vi "Error.Case Redirect on Error.vi"(7 "Error Case":string="Done", 10 "error in":errorcluster, 11 "Next Case":string) -> (3 "Next Case Out":string)   [LabVIEW 2018]
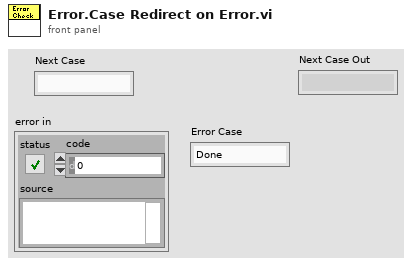
[diagram p1: front panel]
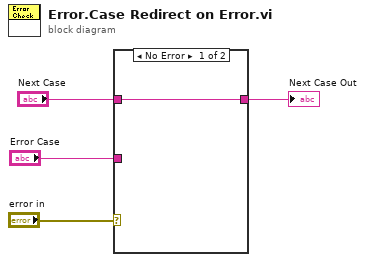
[diagram p0: block diagram]
diagram:
  n1 = case shown="No Error" "error in" {
    tunnel: "Next Case" -> [w5 _]
    tunnel: [w5 w6] -> w2
    tunnel: "Error Case" -> [_ w6]
    frame No Error {
    }
    frame Error {
    }
  }
  "Next Case Out" <- w2
